vi "Load Search  File.vi"(11 "Select Address File           --------------------------->":path) -> (3 "sorted array":string[](array[string]))   [LabVIEW 2020]
uses:
  89d11ad4-5929-3fee-a0be-4eb14e53d83f.vi
  <vilib>/Comparison/Less/Less Functor/Less Functor.lvclass
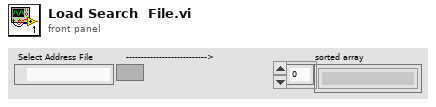
[diagram p1: front panel]
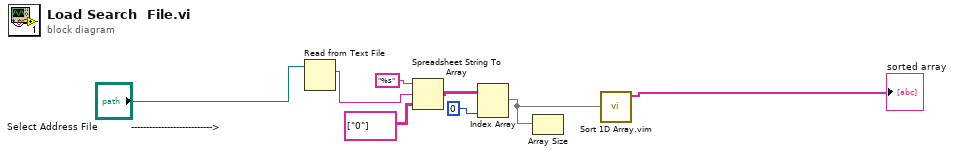
[diagram p0: block diagram]
diagram:
  n1 = Read from Text File(file (use dialog)="Select Address File           --------------------------->") -> (text=w5:string)  [unwired: 3 in, 3 out]
  n2 = Spreadsheet String To Array(format string="%s", spreadsheet string=w5, array type (2D Dbl)=string[][] [["0"]] ("appended array")) -> (array=w4:string[][])  [unwired: 1 in]
  n3 = Index Array(array=w4, index (col)=0 ("disabled index (col)")) -> (element=w6:string[])  [unwired: 1 in]
  n4 = Array Size(array=w6) -> ()  [unwired: 1 out]
  n5 = call "Sort 1D Array.vim"("unsorted array"=w6) -> ("sorted array"=→"sorted array":string[])  [unwired: 10 in]
